vi "Compiler RPN.VI"(1 "string":string) -> (0 "result as string":string)   [LabVIEW 2014, in "NI_Gmath.lvlib"]
uses:
  NI_Gmath.lvlib
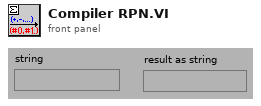
[diagram p1: front panel]
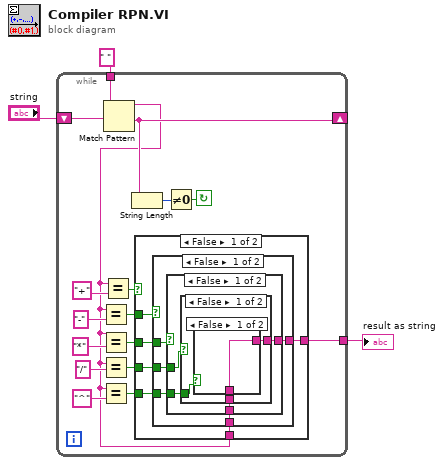
[diagram p0: block diagram]
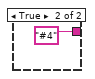
[diagram p2: hidden frame]
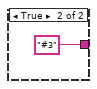
[diagram p3: hidden frame]
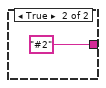
[diagram p4: hidden frame]
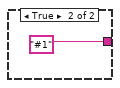
[diagram p5: hidden frame]
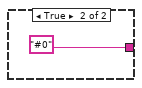
[diagram p6: hidden frame]
diagram:
  n1 = while {
    tunnel: [w4] -> w1
    tunnel: " " -> [w20]
    shift-left: "string" -> [w19]
    shift-right: [w18] -> _
    stop <- w16 continue-if-true
    n2 = Match Pattern(string=w19, regular expression=w20) -> (before substring=w5:string, after substring=w18:string)  [unwired: 1 in, 2 out]
    n3 = Equal?(x=w5, y="-") -> (x = y?=w9:bool)
    n4 = Equal?(x=w5, y="*") -> (x = y?=w8:bool)
    n5 = Equal?(x=w5, y="/") -> (x = y?=w7:bool)
    n6 = Equal?(x=w5, y="^") -> (x = y?=w6:bool)
    n7 = Equal?(x=w5, y="+") -> (x = y?=w14:bool)
    n8 = String Length(string=w18) -> (length=w17:i32)
    n9 = case shown="False" w14 {
      tunnel: w9 -> [w26 _]
      tunnel: w8 -> [w25 _]
      tunnel: w7 -> [w24 _]
      tunnel: w6 -> [w23 _]
      tunnel: [w22 "#0"] -> w4
      tunnel: w5 -> [w21 _]
      frame False {
        n10 = case shown="False" w26 {
          tunnel: w25 -> [w31 _]
          tunnel: w24 -> [w30 _]
          tunnel: w23 -> [w29 _]
          tunnel: [w28 "#1"] -> w22
          tunnel: w21 -> [w27 _]
          frame False {
            n11 = case shown="False" w31 {
              tunnel: w30 -> [w35 _]
              tunnel: w29 -> [w34 _]
              tunnel: [w33 "#2"] -> w28
              tunnel: w27 -> [w32 _]
              frame False {
                n12 = case shown="False" w35 {
                  tunnel: w34 -> [w38 _]
                  tunnel: [w37 "#3"] -> w33
                  tunnel: w32 -> [w36 _]
                  frame False {
                    n13 = case shown="False" w38 {
                      tunnel: [w39 "#4"] -> w37
                      tunnel: w36 -> [w39 _]
                      frame False {
                      }
                      frame True {
                      }
                    }
                  }
                  frame True {
                  }
                }
              }
              frame True {
              }
            }
          }
          frame True {
          }
        }
      }
      frame True {
      }
    }
    n14 = Not Equal To 0?(x=w17) -> (x != 0?=w16:bool)
  }
  "result as string" <- w1
